vi "MenuOptions.vi"(8 "error in":errorcluster, 9 "VI ref":refnum<vi>, 11 "menu ref in":refnum<k9>) -> (0 "error out":errorcluster, 3 "menu ref out":refnum<k9>)   [LabVIEW 2015, in "Configuration Tool.lvlib"]
doc: "This VI configures the application menu options. If you need aditional menu items add them in this VI."
uses:
  Configuration Tool.lvlib
  <vilib>/Utility/miscctls.llb/LVMenuShortCut.ctl
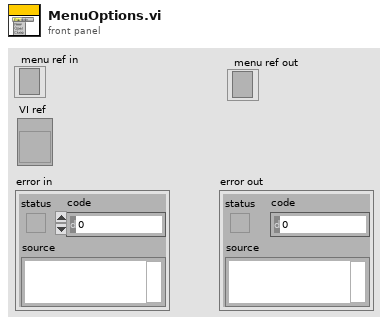
[diagram p1: front panel]
types:
  T1 = typedef "LVMenuShortCut.ctl" = cluster{"Include Shift Key?":bool, "Include Ctrl Key?":bool, "Shortcut Key":string}
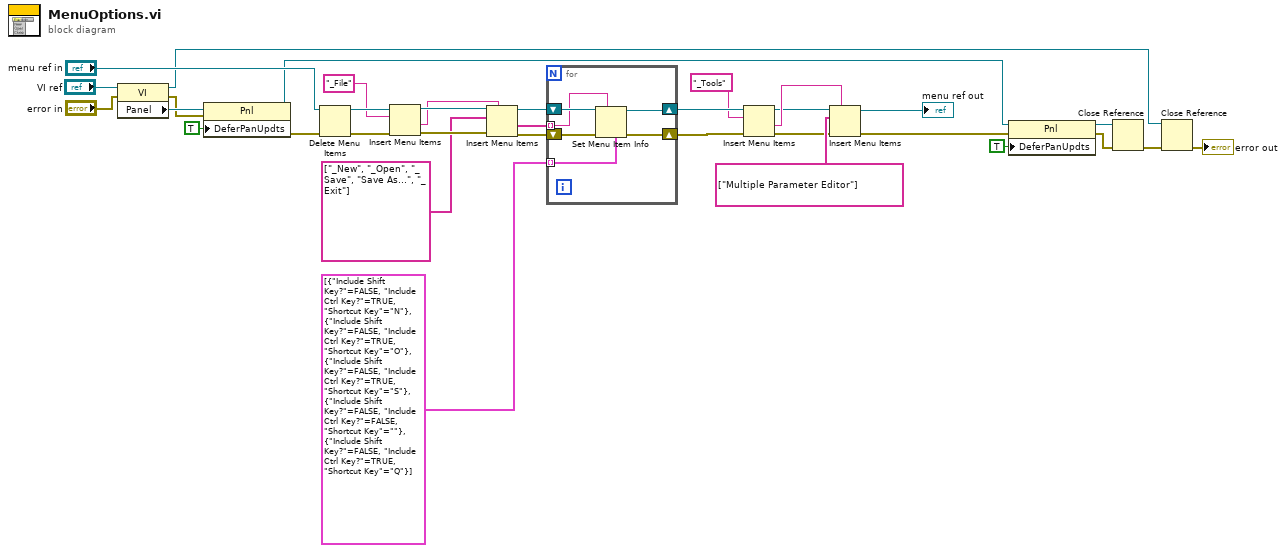
[diagram p0: block diagram]
diagram:
  n1 = property class="VI"(reference="VI ref", error in="error in") -> (reference out=w13:refnum<vi>, error out=w9:errorcluster, "Panel"=w12:refnum<vi>)
  n2 = property class="Pnl"(reference=w12, error in=w9, "DeferPanUpdts"=TRUE ("Defer Panel Updates")) -> (reference out=w5:refnum<vi>, error out=w8:errorcluster)
  n3 = Delete Menu Items(6:w8, 9:"menu ref in") -> (0:w29:errorcluster, 3:w33:refnum<k9>)  [unwired: 2 in]
  n4 = Insert Menu Items(6:w29, 8:"_File", 9:w33) -> (0:w28:errorcluster, 1:w30:string, 3:w31:refnum<k9>)  [unwired: 3 in]
  n5 = Insert Menu Items(5:w30, 6:w28, 8:string[] ["_New", "_Open", "_Save", "Save As...", "_Exit"] ("item names"), 9:w31) -> (0:w25:errorcluster, 1:w24:string[], 3:w26:refnum<k9>)  [unwired: 2 in]
  n6 = for {
    shift-right: [w38] -> w21
    shift-left: w26 -> [w40]
    tunnel: w24 -> [w37] mode=indexing
    tunnel: T1[] [{"Include Shift Key?"=FALSE, "Include Ctrl Key?"=TRUE, "Shortcut Key"="N"}, {"Include Shift Key?"=FALSE, "Include Ctrl Key?"=TRUE, "Shortcut Key"="O"}, {"Include Shift Key?"=FALSE, "Include Ctrl Key?"=TRUE, "Shortcut Key"="S"}, {"Include Shift Key?"=FALSE, "Include Ctrl Key?"=FALSE, "Shortcut Key"=""}, {"Include Shift Key?"=FALSE, "Include Ctrl Key?"=TRUE, "Shortcut Key"="Q"}] -> [w35] mode=indexing
    shift-right: [w36] -> w20
    shift-left: w25 -> [w39]
    n7 = Set Menu Item Info(4:w35, 7:w37, 8:w39, 11:w40) -> (0:w36:errorcluster, 3:w38:refnum<k9>)  [unwired: 3 in]
  }
  n8 = Insert Menu Items(6:w20, 8:"_Tools", 9:w21) -> (0:w17:errorcluster, 1:w19:string, 3:w16:refnum<k9>)  [unwired: 3 in]
  n9 = Insert Menu Items(5:w19, 6:w17, 8:string[] ["Multiple Parameter Editor"] ("item names"), 9:w16) -> (0:w6:errorcluster, 3:→"menu ref out":refnum<k9>)  [unwired: 2 in, 1 out]
  n10 = property class="Pnl"(reference=w5, error in=w6, "DeferPanUpdts"=TRUE ("Defer Panel Updates")) -> (reference out=w4:refnum<vi>, error out=w3:errorcluster)
  n11 = Close Reference(reference=w4, error in (no error)=w3) -> (error out=w2:errorcluster)
  n12 = Close Reference(reference=w13, error in (no error)=w2) -> (error out=→"error out":errorcluster)
